vi "02-sense-dashboard.vi"() -> ()   [LabVIEW 2026]
uses:
  <vilib>/Utility/error.llb/Trim Whitespace One-Sided.vi
panel:
  in  "stop":bool
  out "XY Graph":cluster{"X":dbl, "Y":dbl}[](graph)
  out "Error":bool
  out "Status":bool
  out "AQI":dbl
  out "UV":dbl
  out "Temperatrue":dbl
  out "Humidity":dbl
  out "Soilinfg Ratio":dbl(knob) scale=0.0..10.0
  out "Panel 3 Efficiency 2":dbl(knob) scale=0.0..100.0
  out "Panel 2 Efficiency":dbl(knob) scale=0.0..100.0
  out "Panel 1 Efficiency":dbl(knob) scale=0.0..100.0
  out "Tank":dbl(slide) scale=0.0..100.0
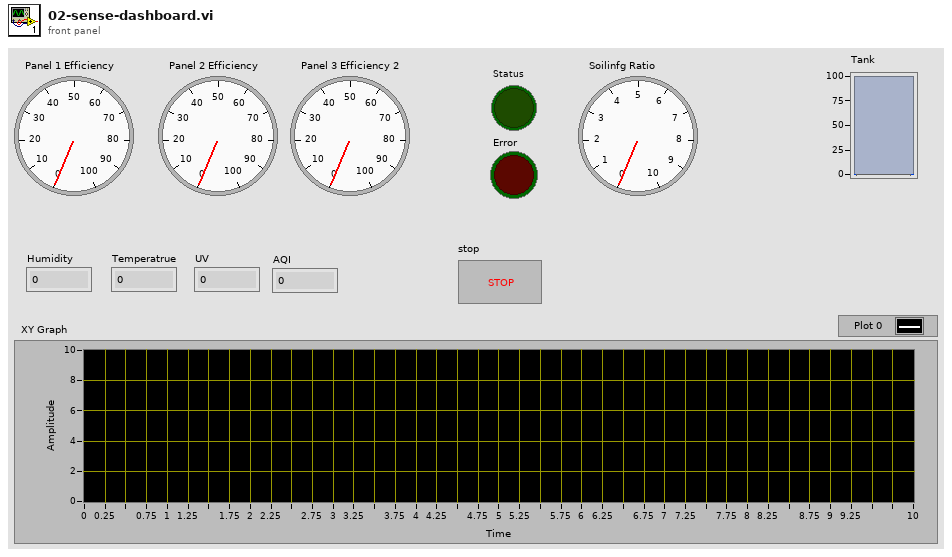
[diagram p1: front panel]
types:
  T1 = cluster{"panel_efficiency":dbl[], "soiling_ratio":dbl, "humidity":dbl, "temperature":dbl, "uv":dbl, "aqi":i32, "battery":dbl, "status_ok":dbl, "error":dbl}
  T2 = enum16{"Standard", "Buffered", "CRLF", "Immediate"}
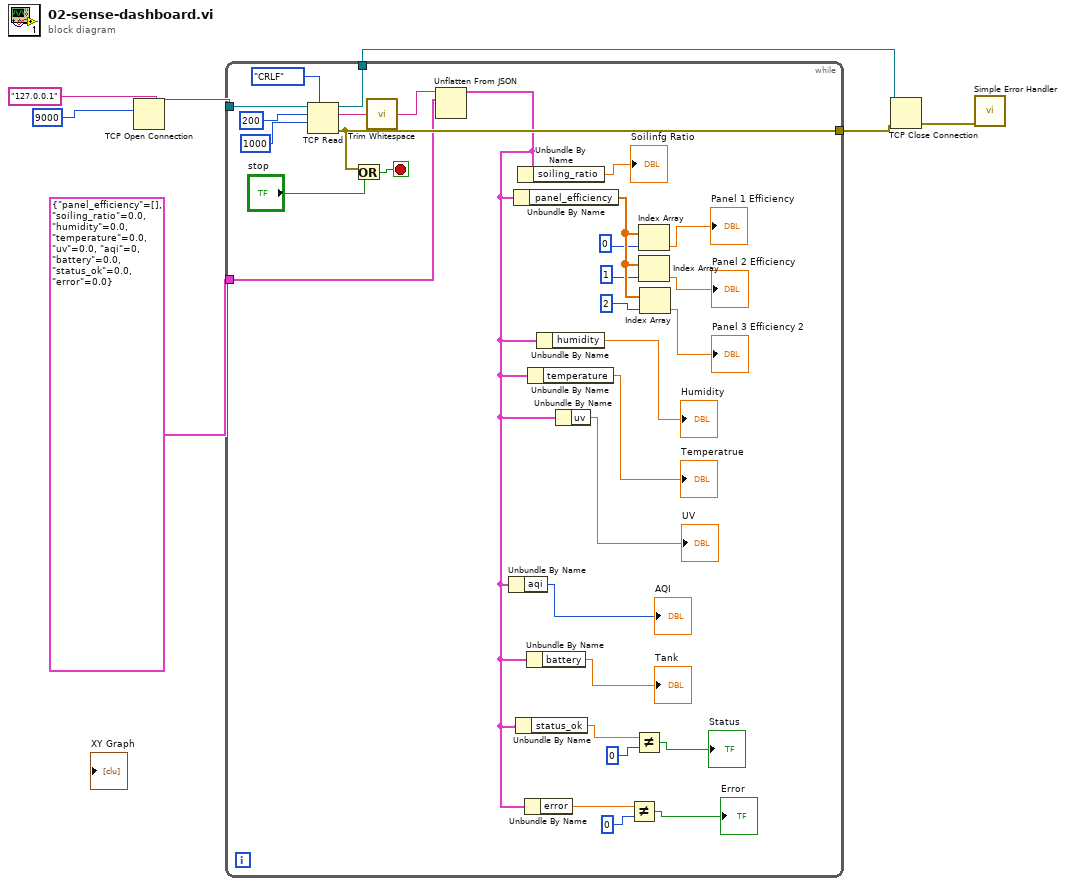
[diagram p0: block diagram]
diagram:
  n1 = TCP Open Connection(address="127.0.0.1", remote port or service name=9000) -> (connection ID=w5:refnum<k5>)  [unwired: 3 in, 1 out]
  n2 = while {
    tunnel: w5 -> [w38]
    tunnel: [w33] -> w3
    tunnel: [w32] -> w2
    tunnel: T1 {"panel_efficiency"=[], "soiling_ratio"=0.0, "humidity"=0.0, "temperature"=0.0, "uv"=0.0, "aqi"=0, "battery"=0.0, "status_ok"=0.0, "error"=0.0} -> [w28]
    stop <- w31 stop-if-true
    n3 = TCP Read(connection ID=w38, bytes to read=200, 7:T2."CRLF" ("mode (standard)"), 9:1000) -> (connection ID out=w33:refnum<k5>, data out=w34:string, error out=w32:errorcluster)  [unwired: 1 in]
    n4 = Or(x=w32, y="stop") -> (x .or. y?=w31:bool)
    n5 = call <vilib>:"Trim Whitespace.vi"("string"=w34) -> ("trimmed string"=w29:string)  [unwired: 1 in]
    n6 = Unflatten From JSON(JSON string=w29, type and defaults=w28) -> (value=w14:T1)  [unwired: 5 in, 1 out]
    n7 = Unbundle By Name(w14) -> ("aqi"=→"AQI":i32)
    n8 = Unbundle By Name(w14) -> ("panel_efficiency"=w26:dbl[])
    n9 = Unbundle By Name(w14) -> ("status_ok"=w13:dbl)
    n10 = Unbundle By Name(w14) -> ("soiling_ratio"=→"Soilinfg Ratio":dbl)
    n11 = Unbundle By Name(w14) -> ("error"=w10:dbl)
    n12 = Unbundle By Name(w14) -> ("battery"=→"Tank":dbl)
    n13 = Unbundle By Name(w14) -> ("temperature"=→"Temperatrue":dbl)
    n14 = Unbundle By Name(w14) -> ("humidity"=→"Humidity":dbl)
    n15 = Unbundle By Name(w14) -> ("uv"=→"UV":dbl)
    n16 = Not Equal?(x=w10, y=0) -> (x != y?=→"Error":bool)
    n17 = Not Equal?(x=w13, y=0) -> (x != y?=→"Status":bool)
    n18 = Index Array(array=w26, index=0) -> (element=→"Panel 1 Efficiency":dbl)
    n19 = Index Array(array=w26, index=1) -> (element=→"Panel 2 Efficiency":dbl)
    n20 = Index Array(array=w26, index=2) -> (element=→"Panel 3 Efficiency 2":dbl)
  }
  n21 = TCP Close Connection(connection ID=w3, error in (no error)=w2) -> (error out=w4:errorcluster)  [unwired: 1 in, 1 out]
  n22 = call <vilib>:"Simple Error Handler.vi"("error in (no error)"=w4) -> ()  [unwired: 4 in, 5 out]
